vi "Initialize.vi"(8 "error in (no error)":errorcluster, 10 "DAQ Configuration":T1={"Shutters"=[], "fluidics trigger line"="Dev1/port1/line1", "camera trigger line"="", "COM Port"="COM3", "Device type"=enum."NI DAQ"}, 11 "Synchronization Device in":refnum<class "Sync Device.lvclass">) -> (0 "error out":errorcluster, 3 "Synchronization Device out":refnum<class "Sync Device.lvclass">, 4 "Trigger Jitter (ms)":dbl)   [LabVIEW 2023, in "Sync Device.lvlib" / "Sync Device.lvclass"]
uses:
  Sync Device.lvclass
  Resources/Type Defs/DAQ Configuration.ctl
  Resources/Type Defs/Shutter Configuration.ctl
  Resources/Type Defs/Sync Device Type.ctl
  Sync Device.lvclass/Sync Device.ctl
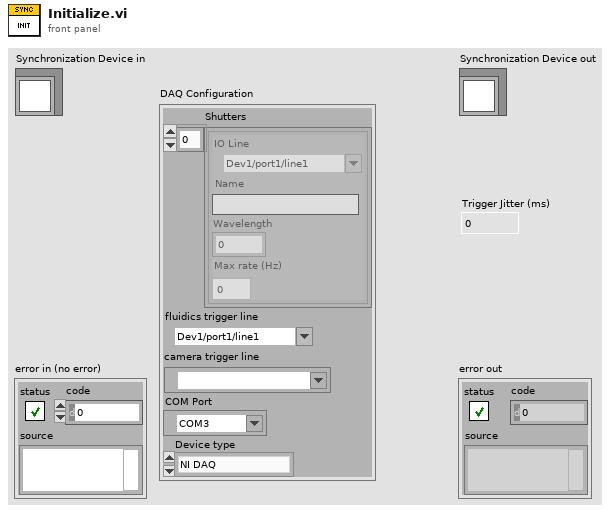
[diagram p1: front panel]
types:
  T1 = typedef "DAQ Configuration.ctl" = cluster{"Shutters":T2[], "fluidics trigger line":tag, "camera trigger line":tag, "COM Port":refnum<visa-resource-name>, "Device type":T3}
  T2 = typedef "Shutter Configuration.ctl" = cluster{"IO Line":tag, "Name":string, "Wavelength":u16, "Max rate (Hz)":dbl}
  T3 = typedef "Sync Device Type.ctl" = enum16{"Disabled", "NI DAQ", "Arduino DAQ"}
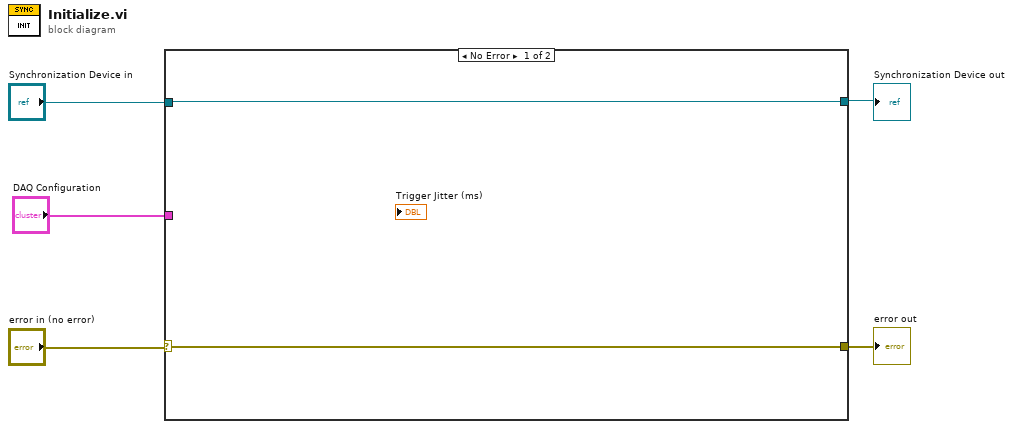
[diagram p0: block diagram]
diagram:
  n1 = case shown="No Error" "error in (no error)" {
    selector: "error in (no error)" -> [w7 w9]
    tunnel: [w7 w9] -> w4
    tunnel: [w6 w8] -> w2
    tunnel: "Synchronization Device in" -> [w6 w8]
    tunnel: "DAQ Configuration" -> [_ _]
    frame No Error {
    }
    frame Error {
    }
  }
  "error out" <- w4
  "Synchronization Device out" <- w2
